vi "notify user TRA problem.vi"(0 "At least 1 out of range":bool) -> ()   [LabVIEW 2011]
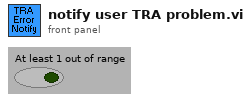
[diagram p1: front panel]
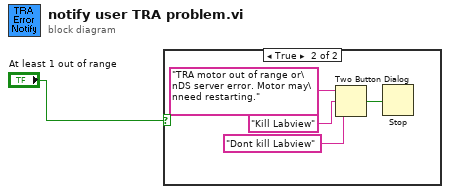
[diagram p0: block diagram]
diagram:
  n1 = case shown="True" "At least 1 out of range" {
    frame False {
    }
    frame True {
      n2 = Two Button Dialog(message="TRA motor out of range or\nDS server error. Motor may\nneed restarting.", 1:"Dont kill Labview" ("F button name (\"Cancel\")"), 2:"Kill Labview" ("T button name (\"OK\")")) -> (T button?=w2:bool)
      n3 = Stop(stop? (T)=w2) -> ()
    }
  }
